vi "Conv_POSE_SI_Eng.vi"(11 "Err Pose in SI":T1) -> (3 "Err Pose out ENG":T1)   [LabVIEW 2019, in "Trajectory_Library.lvlib"]
doc: "Convert POSE from Meters, Radians to Feet, Degrees. (This is really only for external use. All the internal routines use meters and radians.)"
uses:
  Trajectory_Library.lvlib
  TRANSLATION2D.ctl
  ROTATION2D.ctl
  POSE2D.ctl
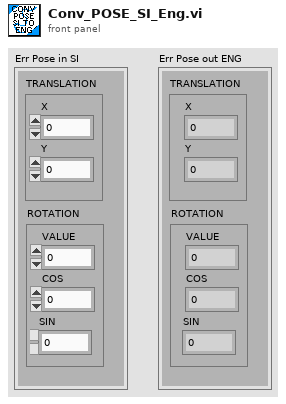
[diagram p1: front panel]
types:
  T1 = typedef "Trajectory_Library.lvlib/POSE2D.ctl" = cluster{"TRANSLATION":T2, "ROTATION":T3}
  T2 = typedef "Trajectory_Library.lvlib/TRANSLATION2D.ctl" = cluster{"X":dbl, "Y":dbl}
  T3 = typedef "Trajectory_Library.lvlib/ROTATION2D.ctl" = cluster{"VALUE":dbl, "COS":dbl, "SIN":dbl}
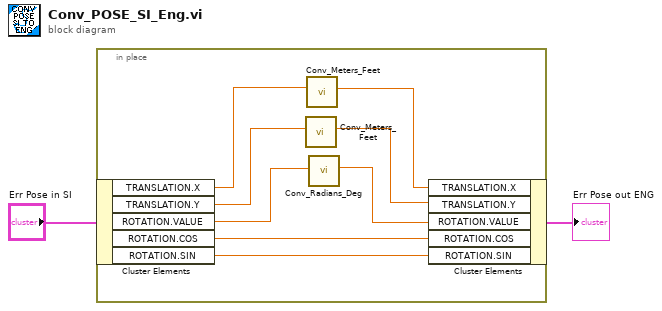
[diagram p0: block diagram]
diagram:
  n1 = in-place {
    n2 = in-place-cluster #1("Err Pose in SI") -> ("TRANSLATION.X"=w10:dbl, "TRANSLATION.Y"=w8:dbl, "ROTATION.VALUE"=w6:dbl, "ROTATION.COS"=w4:dbl, "ROTATION.SIN"=w3:dbl)
    n3 = call "Conv_Meters_Feet.vi"("Meters"=w8) -> ("Feet"=w7:dbl)  [unwired: 10 in]
    n4 = call "Conv_Meters_Feet.vi"("Meters"=w10) -> ("Feet"=w9:dbl)  [unwired: 10 in]
    n5 = call "Conv_Radians_Deg.vi"("Radians"=w6) -> ("Degrees"=w5:dbl)  [unwired: 10 in]
    n6 = in-place-cluster #1("TRANSLATION.X"=w9, "TRANSLATION.Y"=w7, "ROTATION.VALUE"=w5, "ROTATION.COS"=w4, "ROTATION.SIN"=w3) -> (→"Err Pose out ENG":T1)
  }
